vi "get waveform - source.vi"(8 "error in (no error)":errorcluster caption="에러 입력(에러 없음)", 11 "WAV File 입력":refnum<class "WAV File.lvclass">) -> (0 "error out":errorcluster caption="에러 출력", 2 "waveform":waveform(dbl), 3 "WAV File 출력":refnum<class "WAV File.lvclass">)   [LabVIEW 2020, in "WAV File.lvclass"]
uses:
  WAV File.lvclass
  WAV File.lvclass/WAV File.ctl
  Accessors/Read sound format.vi
  Accessors/Read normalize.vi
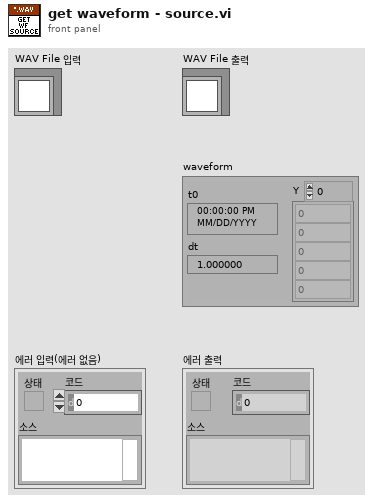
[diagram p1: front panel]
types:
  T1 = typedef "Sound Data Format.ctl" = cluster{"sample rate (S/s)":dbl, "number of channels":i32, "bits per sample":i32}
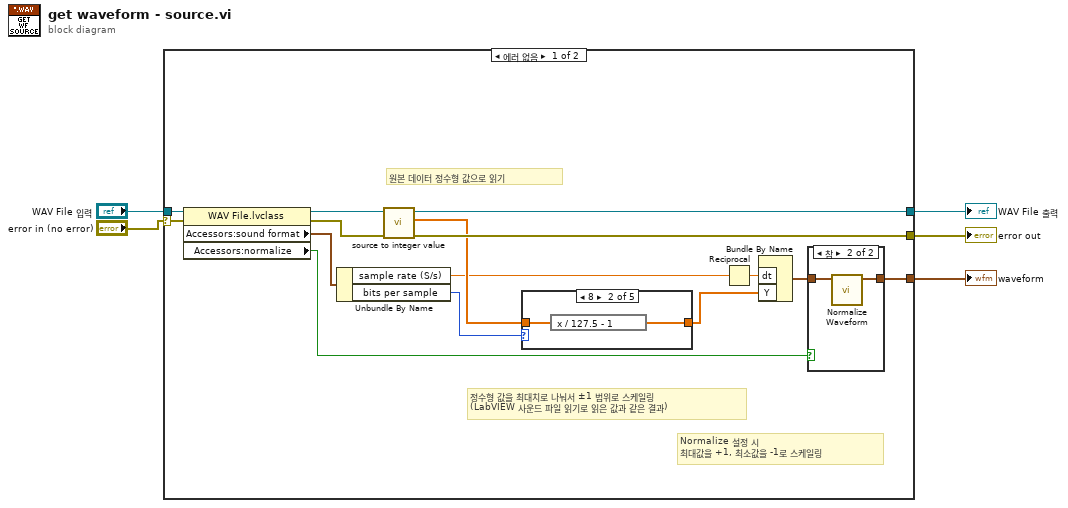
[diagram p0: block diagram]
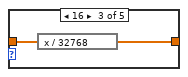
[diagram p4: hidden frame]
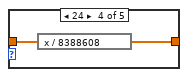
[diagram p5: hidden frame]
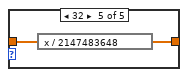
[diagram p6: hidden frame]
diagram:
  n1 = case shown="에러 없음" "error in (no error)" {
    selector: "error in (no error)" -> [w19 w33]
    tunnel: [w15 w33] -> w1
    tunnel: "WAV File 입력" -> [w20 w32]
    tunnel: [w13 w32] -> w4
    tunnel: [w7 _] -> w3
    frame No Error {
      # "원본 데이터 정수형 값으로 읽기"
      # "Normalize 설정 시\n최대값을 +1, 최소값을 -1로 스케일링"
      # "정수형 값을 최대치로 나눠서 ±1 범위로 스케일링\n(LabVIEW 사운드 파일 읽기로 읽은 값과 같은 결과)"
      n2 = property class="WAV File.lvclass"(reference=w20, error in=w19) -> (reference out=w14:refnum<class "WAV File.lvclass">, error out=w16:errorcluster, "Accessors:sound format"=w12:T1, "Accessors:normalize"=w6:bool)
      n3 = Unbundle By Name(w12) -> ("sample rate (S/s)"=w8:dbl, "bits per sample"=w9:i32)
      n4 = call-dynamic "source to integer value.vi"("error in (no error)"=w16, "WAV File 입력"=w14) -> ("error out"=w15:errorcluster, "integer value"=w10:dbl[], "WAV File 출력"=w13:refnum<class "WAV File.lvclass">)  [unwired: 7 in]
      n5 = case shown="8" w9 {
        tunnel: [_ w25 w27 w29 w31] -> w11
        tunnel: w10 -> [_ w24 w26 w28 w30]
        frame 0, Default {
        }
        frame 8 {
          n6 = expression code="x / 127.5 - 1"(w24) -> (w25:dbl[])
        }
        frame 16 {
          n7 = expression code="x / 32768"(w26) -> (w27:dbl[])
        }
        frame 24 {
          n8 = expression code="x / 8388608"(w28) -> (w29:dbl[])
        }
        frame 32 {
          n9 = expression code="x / 2147483648"(w30) -> (w31:dbl[])
        }
      }
      n10 = Reciprocal(x=w8) -> (1/x=w18:dbl)
      n11 = Bundle By Name("dt"=w18, "Y"=w11) -> (w17:waveform(dbl))  [unwired: 1 in]
      n12 = case shown="참" w6 {
        tunnel: w17 -> [w21 w23]
        tunnel: [w21 w22] -> w7
        frame False {
        }
        frame True {
          n13 = call <vilib>:"Normalize Waveform.vi"("waveform in"=w23) -> ("normalized waveform"=w22:waveform(dbl))  [unwired: 7 in, 3 out]
        }
      }
    }
    frame Error {
    }
  }
  "error out" <- w1
  "WAV File 출력" <- w4
  "waveform" <- w3
